vi "main.vi"() -> ()   [LabVIEW 2013]
uses:
  WasRun.lvclass
panel:
  out "was run 3":bool
  in  "was run 2":bool
  out "was run":bool
  out "error out":errorcluster
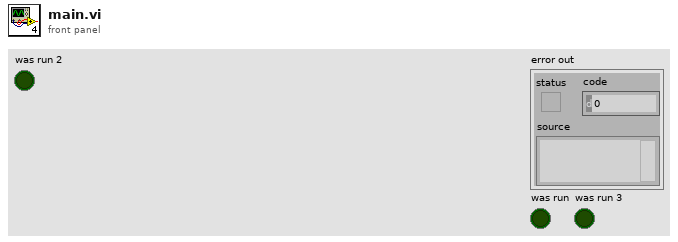
[diagram p1: front panel]
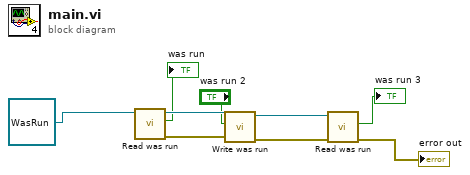
[diagram p0: block diagram]
diagram:
  n1 = call-dynamic "Read was run.vi"("WasRun in"=refnum<class "WasRun.lvclass"> refnum ("WasRun.lvclass")) -> ("error out"=w8:errorcluster, "was run"=→"was run":bool, "WasRun out"=w6:refnum<class "WasRun.lvclass">)  [unwired: 8 in]
  n2 = call-dynamic "Write was run.vi"("error in (no error)"=w8, "was run"="was run 2", "WasRun in"=w6) -> ("error out"=w7:errorcluster, "WasRun out"=w5:refnum<class "WasRun.lvclass">)  [unwired: 7 in]
  n3 = call-dynamic "Read was run.vi"("error in (no error)"=w7, "WasRun in"=w5) -> ("error out"=→"error out":errorcluster, "was run"=→"was run 3":bool)  [unwired: 7 in, 1 out]
